vi "SSP - set value STR.vi"(8 "error in (no error)":errorcluster, 11 "JSON string":string) -> (0 "error out":errorcluster, 3 "value":string)   [LabVIEW 2020, in "ui-testing.lvlib"]
doc: "copyright: Thomas Zilliox©"
uses:
  ui-testing.lvlib
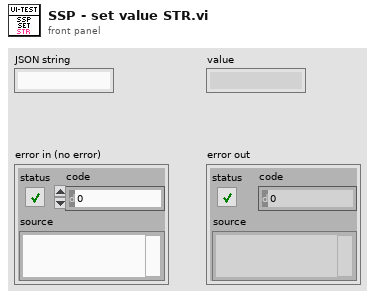
[diagram p1: front panel]
types:
  T1 = cluster{"control":string, "subpanel":string, "subsubpanel":string, "value":string}
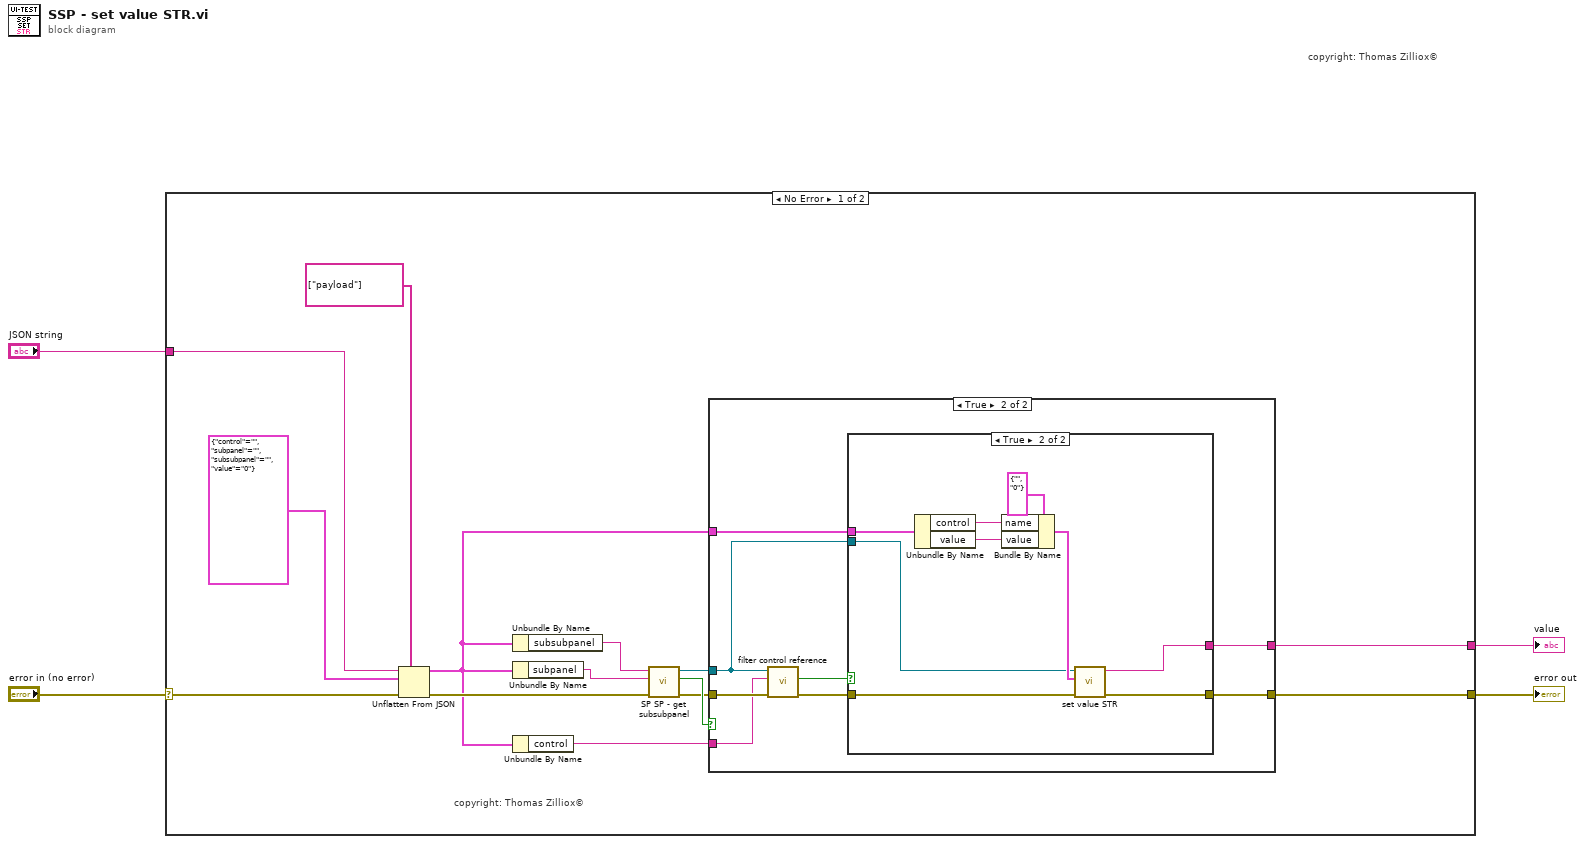
[diagram p0: block diagram]
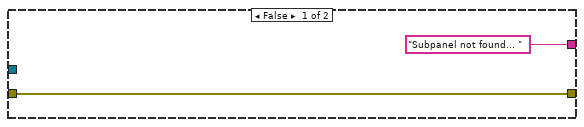
[diagram p2: hidden frame]
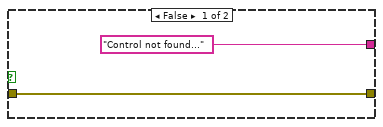
[diagram p3: hidden frame]
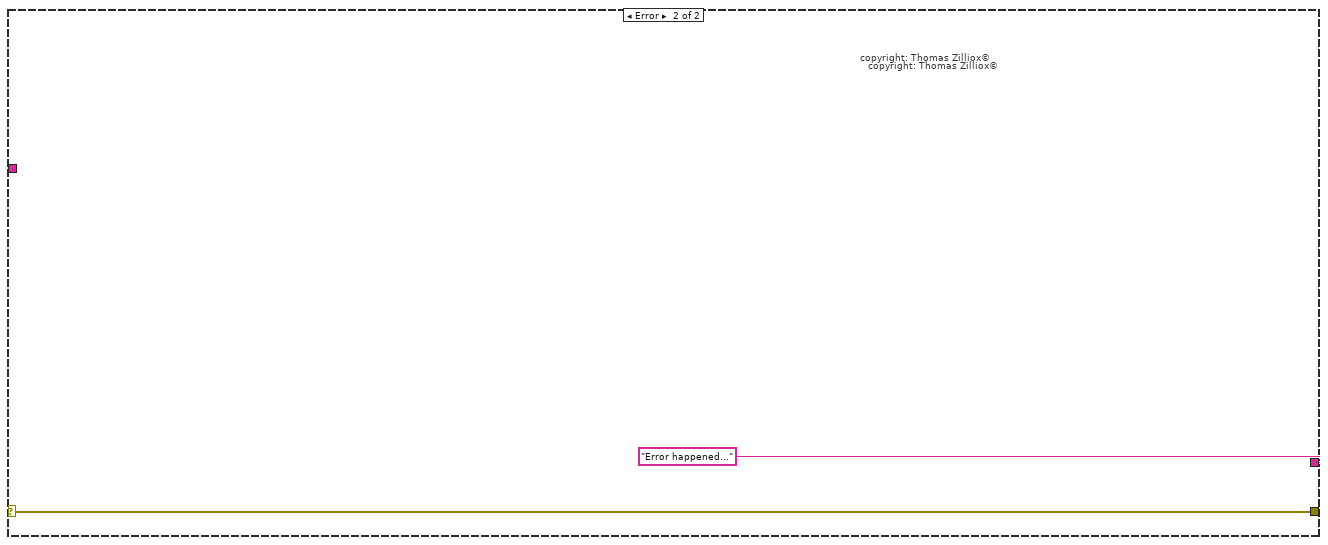
[diagram p4: hidden frame]
diagram:
  # "copyright: Thomas Zilliox©"
  n1 = case shown="No Error" "error in (no error)" {
    selector: "error in (no error)" -> [w14 w41]
    tunnel: "JSON string" -> [w16 _]
    tunnel: [w15 w41] -> w3
    tunnel: [w13 "Error happened..."] -> w1
    frame No Error {
      # "copyright: Thomas Zilliox©"
      n2 = Unflatten From JSON(path=string[] ["payload"], JSON string=w16, type and defaults=T1 {"control"="", "subpanel"="", "subsubpanel"="", "value"="0"}, error in (no error)=w14) -> (value=w6:T1, error out=w17:errorcluster)  [unwired: 3 in]
      n3 = Unbundle By Name(w6) -> ("subsubpanel"=w5:string)
      n4 = Unbundle By Name(w6) -> ("subpanel"=w12:string)
      n5 = Unbundle By Name(w6) -> ("control"=w9:string)
      n6 = call "SP SP - get subsubpanel.vi"("error in (no error)"=w17, "subpanel"=w12, "subsubpanel"=w5) -> ("error out"=w7:errorcluster, "SubSubPanel found"=w8:bool, "SubSubPanel VI"=w10:refnum<vi>)  [unwired: 5 in, 1 out]
      n7 = case shown="True" w8 {
        tunnel: [w20 w28] -> w15
        tunnel: w10 -> [_ w25]
        tunnel: w7 -> [w20 w24]
        tunnel: w9 -> [_ w23]
        tunnel: ["Subpanel not found... " ("result string") w27] -> w13
        tunnel: w6 -> [_ w26]
        frame False {
        }
        frame True {
          n8 = call "filter control reference.vi"("error in (no error)"=w24, "Control label"=w23, "VI (Caller)"=w25) -> ("error out"=w21:errorcluster, "Control found"=w22:bool)  [unwired: 6 in, 1 out]
          n9 = case shown="True" w22 {
            tunnel: w21 -> [w30 w33]
            tunnel: [w30 w31] -> w28
            tunnel: ["Control not found..." ("result string") w32] -> w27
            tunnel: w26 -> [_ w35]
            tunnel: w25 -> [_ w34]
            frame False {
            }
            frame True {
              n10 = Unbundle By Name(w35) -> ("control"=w36:string, "value"=w37:string)
              n11 = Bundle By Name(cluster=cluster{"name":string, "value":string} {"name"="", "value"="0"} ("Payload"), "name"=w36, "value"=w37) -> (w38:cluster{"name":string, "value":string})
              n12 = call "set value STR.vi"("error in (no error)"=w33, "Payload"=w38, "VI Ref"=w34) -> ("error out"=w31:errorcluster, "return value"=w32:string)  [unwired: 7 in]
            }
          }
        }
      }
    }
    frame Error {
      # "copyright: Thomas Zilliox©"
      # "copyright: Thomas Zilliox©"
    }
  }
  "error out" <- w3
  "value" <- w1
